vi "脉冲生成_基于时间_单脉冲.vi"() -> ()   [LabVIEW 2013]
uses:
  <userlib>/ArtDAQ/_SubVI/ArtDAQ_CreateCOPulseChanTime.vi
  <userlib>/ArtDAQ/_SubVI/ArtDAQ_CfgDigEdgeStartTrig.vi
panel:
  in  "触发模式":enum32{"No Trigger", "DigStartTrig"}(tab)
  in  "触发边沿":i32(ring)=10280 items=["上升"=10280, "下降"=10171]
  in  "触发源":string(combo)="/Dev1/PFI1"
  in  "Stop":bool
  in  "计数器":string="Dev1/ctr0"
  in  "高电平时间":dbl=0.01 format="%0.6f"
  in  "低电平时间":dbl=0.01 caption="高电平时间" format="%0.6f"
  out "错误输出":errorcluster
  # "通道属性"
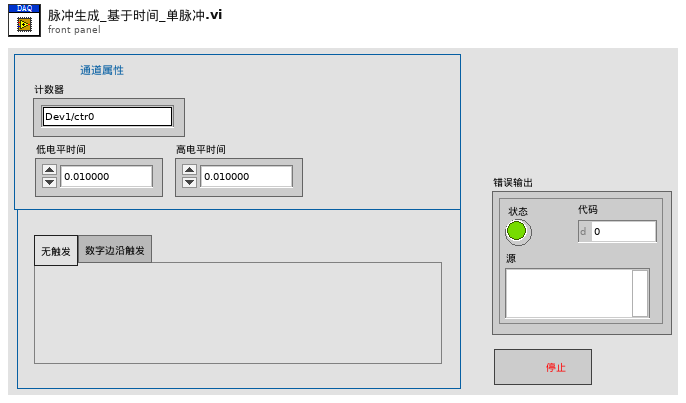
[diagram p1: front panel]
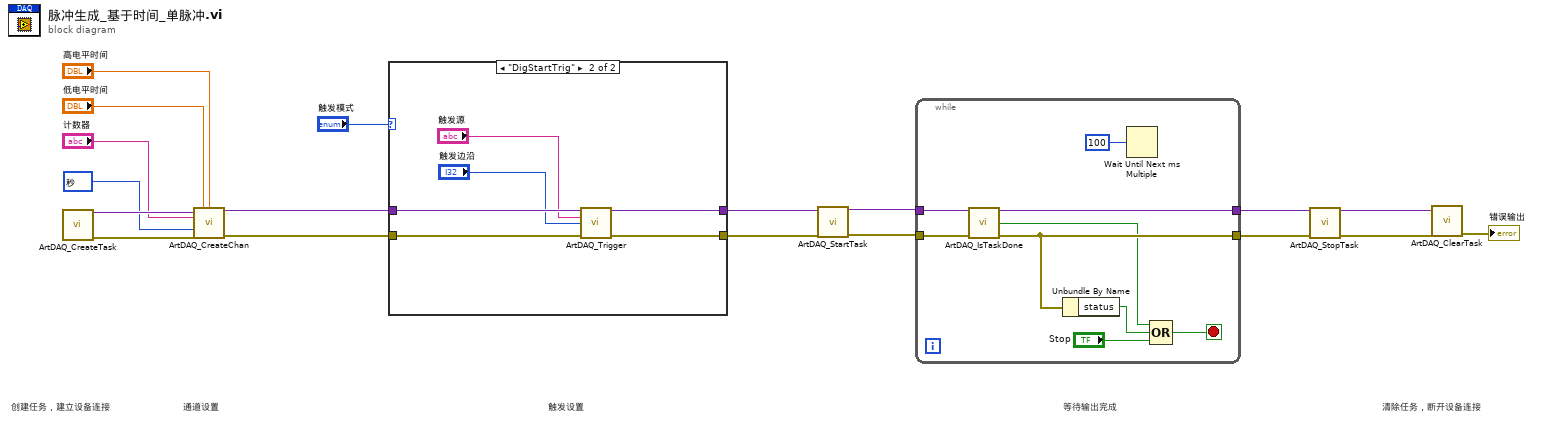
[diagram p0: block diagram]
diagram:
  w3 = 10364 items=["秒"=10364] ("Units")
  # "创建任务，建立设备连接"
  # "通道设置"
  # "触发设置"
  # "等待输出完成"
  # "清除任务，断开设备连接"
  n1 = call <userlib>:"ArtDAQ_CreateTask.vi"() -> ("任务句柄"=w18:variant, "错误输出"=w17:errorcluster)  [unwired: 14 in]
  n2 = call-poly <userlib>:"ArtDAQ_CreateChan.vi"("任务句柄"=w18, "低时间"="低电平时间", "高时间"="高电平时间", "计数器"="计数器", "单位"=w3, "错误输入"=w17) -> ("任务句柄"=w2:variant, "错误输出"=w1:errorcluster)  [unwired: 8 in]
  n3 = case shown="\"DigStartTrig\"" "触发模式" {
    tunnel: w2 -> [w20 w26]
    tunnel: [w20 w25] -> w7
    tunnel: [w19 w24] -> w5
    tunnel: w1 -> [w19 w23]
    frame "No Trigger", Default {
    }
    frame "DigStartTrig" {
      n4 = call-poly <userlib>:"ArtDAQ_Trigger.vi"("任务句柄"=w26, "触发源"="触发源", "边沿"="触发边沿", "错误输入"=w23) -> ("任务句柄"=w25:variant, "错误输出"=w24:errorcluster)  [unwired: 10 in]
    }
  }
  n5 = call <userlib>:"ArtDAQ_StartTask.vi"("任务句柄"=w7, "错误输入"=w5) -> ("任务句柄"=w6:variant, "错误输出"=w4:errorcluster)  [unwired: 12 in]
  n6 = while {
    tunnel: [w35] -> w15
    tunnel: [w34] -> w13
    tunnel: w6 -> [w31]
    tunnel: w4 -> [w30]
    stop <- w29 stop-if-true
    n7 = call <userlib>:"ArtDAQ_IsTaskDone.vi"("任务句柄"=w31, "错误输入"=w30) -> ("任务句柄"=w35:variant, "完成任务？"=w27:bool, "错误输出"=w34:errorcluster)  [unwired: 11 in]
    n8 = Unbundle By Name(w34) -> ("status"=w33:bool)
    n9 = Wait Until Next ms Multiple(millisecond multiple=u32 100 ("毫秒倍数")) -> ()  [unwired: 1 out]
    n10 = Compound Arithmetic op=OR(w27, w33, "Stop") -> (w29:bool)
  }
  n11 = call <userlib>:"ArtDAQ_StopTask.vi"("任务句柄"=w15, "错误输入"=w13) -> ("任务句柄"=w14:variant, "错误输出"=w12:errorcluster)  [unwired: 12 in]
  n12 = call <userlib>:"ArtDAQ_ClearTask.vi"("任务句柄"=w14, "错误输入"=w12) -> ("错误输出"=→"错误输出":errorcluster)  [unwired: 13 in]
